vi "logger_to_event.vi"(8 "error in (no error)":errorcluster) -> (0 "error out":errorcluster, 3 "Time Tagger logger event":refnum<user-event>)   [LabVIEW 2014]
uses:
  SwabianInstruments.TimeTagger
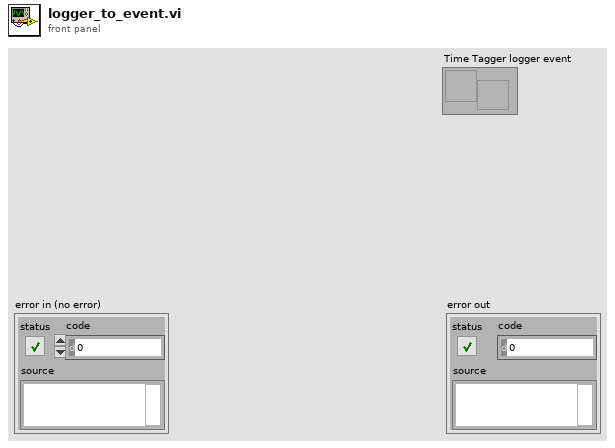
[diagram p1: front panel]
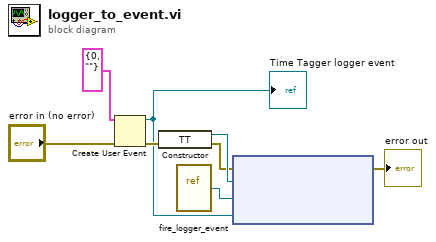
[diagram p0: block diagram]
diagram:
  n1 = Create User Event(user event datatype=cluster{"level":i32, "message":string} {"level"=0, "message"=""} ("Event Data"), error in="error in (no error)") -> (user event=w3:refnum<user-event>, error out=w4:errorcluster)
  "Time Tagger logger event" <- w3
  n2 = constructor class="TT"(error in=w4) -> (reference out=w8:refnum<k24>, error out=w7:errorcluster)  [unwired: 2 in, 1 out]
  n3 = vi-ref "fire_logger_event.vi"() -> ("vi reference"=w2:refnum<vi>)
  n4 = node(w7, w8, w2, w3) -> (→"error out":errorcluster)  [unwired: 1 in, 1 out]
